vi "Main.vi"() -> ()   [LabVIEW 2016]
doc: "The myRIO Project template acquires acceleration data from the onboard accelerometer and displays the changes of acceleration values in a waveform chart."
uses:
  Project Custom Controls/IMU Data Cluster.ctl
  <vilib>/myRIO/Common/Instrument Driver Framework/myRIO v1.0/UART/vis/myRIO v1.0 Close UART.vi
  <vilib>/Instr/_visa.llb/VISA Configure Serial Port (Instr).vi
  <vilib>/myRIO/Common/Instrument Driver Framework/Utilities/vis/FPGA Ref Manager.vi
  <vilib>/myRIO/Common/Instrument Driver Framework/myRIO v1.0/myRIO v1.0 Reset FPGA.vi
  <vilib>/myRIO/Common/Instrument Driver Framework/myRIO v1.0/IRQ/vis/myRIO v1.0 IRQ Info FGV.vi
  <vilib>/myRIO/Common/Instrument Driver Framework/myRIO v1.0/IRQ/vis/myRIO v1.0 Timer IRQ Info FGV.vi
  <vilib>/myRIO/Common/Instrument Driver Framework/myRIO v1.0/IRQ/vis/myRIO v1.0 ISR Agent.vi
  <vilib>/myRIO/Instrument Drivers/Utilities/Utilities.lvlib
panel:
  in  "Roll Gains":T1
  in  "Roll":dbl min=0.0 max=0.08
  in  "Pitch":T1
  in  "Pitch":dbl min=0.0 max=0.08
  in  "Yaw Gains":T1
  in  "Yaw":dbl min=0.0 max=0.08
  in  "Start":bool
  out "Boolean 3":bool
  out "Boolean 2":bool
  out "Loop Iteration":dbl
  out "Waveform Chart":cluster{"Yaw":dbl, "Pitch":dbl, "Roll":dbl}(graph)
  in  "Stop":bool
  out "IMU Data Cluster":T2
  out "Boolean":bool
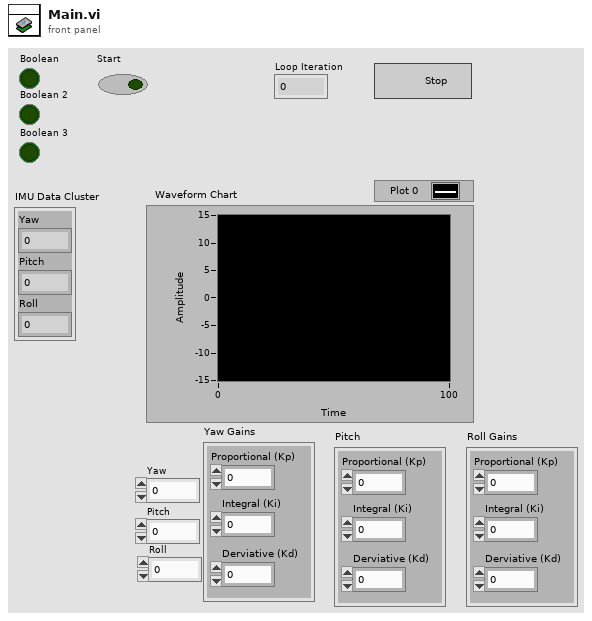
[diagram p1: front panel]
types:
  T1 = cluster{"Proportional (Kp)":dbl, "Integral (Ki)":dbl, "Derviative (Kd)":dbl}
  T2 = typedef "IMU Data Cluster.ctl" = cluster{"Yaw":dbl, "Pitch":dbl, "Roll":dbl}
  T3 = typedef "PWM.lvlib/PWM Reference.ctl" = cluster{"myRIO Reference":T4, "PWM Channels Enum":T8, "PWM Configuration":T9}
  T4 = typedef "myRIO Generic Hardware Reference.ctl" = cluster{"myRIO Model":T5, "myRIO Hardware Reference":T6}
  T5 = typedef "Hardware Version Enum.ctl" = enum16{"Unknown", "myRIO-1900", "myRIO-1950", "roboRIO", "NI ELVIS RIO CM"}
  T6 = typedef "myRIO v1.0 Reference.ctl" = cluster{"Generic FPGA Reference":T7, "Allow multiple opens":bool}
  T7 = typedef "Generic FPGA Reference.ctl" = refnum<k20>
  T8 = typedef "PWM Channels Enum.ctl" = enum16{"Not Connected", "C/PWM0", "C/PWM1", "A/PWM0", "A/PWM1", "A/PWM2", "B/PWM0", "B/PWM1", "B/PWM2", "PWM/PWM0", "PWM/PWM1", "PWM/PWM2", "PWM/PWM3", "PWM/PWM4", "PWM/PWM5", "PWM/PWM6", "PWM/PWM7", "PWM/PWM8", "PWM/PWM9"}
  T9 = typedef "PWM.lvlib/PWM Configuration.ctl" = cluster{"Frequency":dbl, "Duty Cycle":dbl}
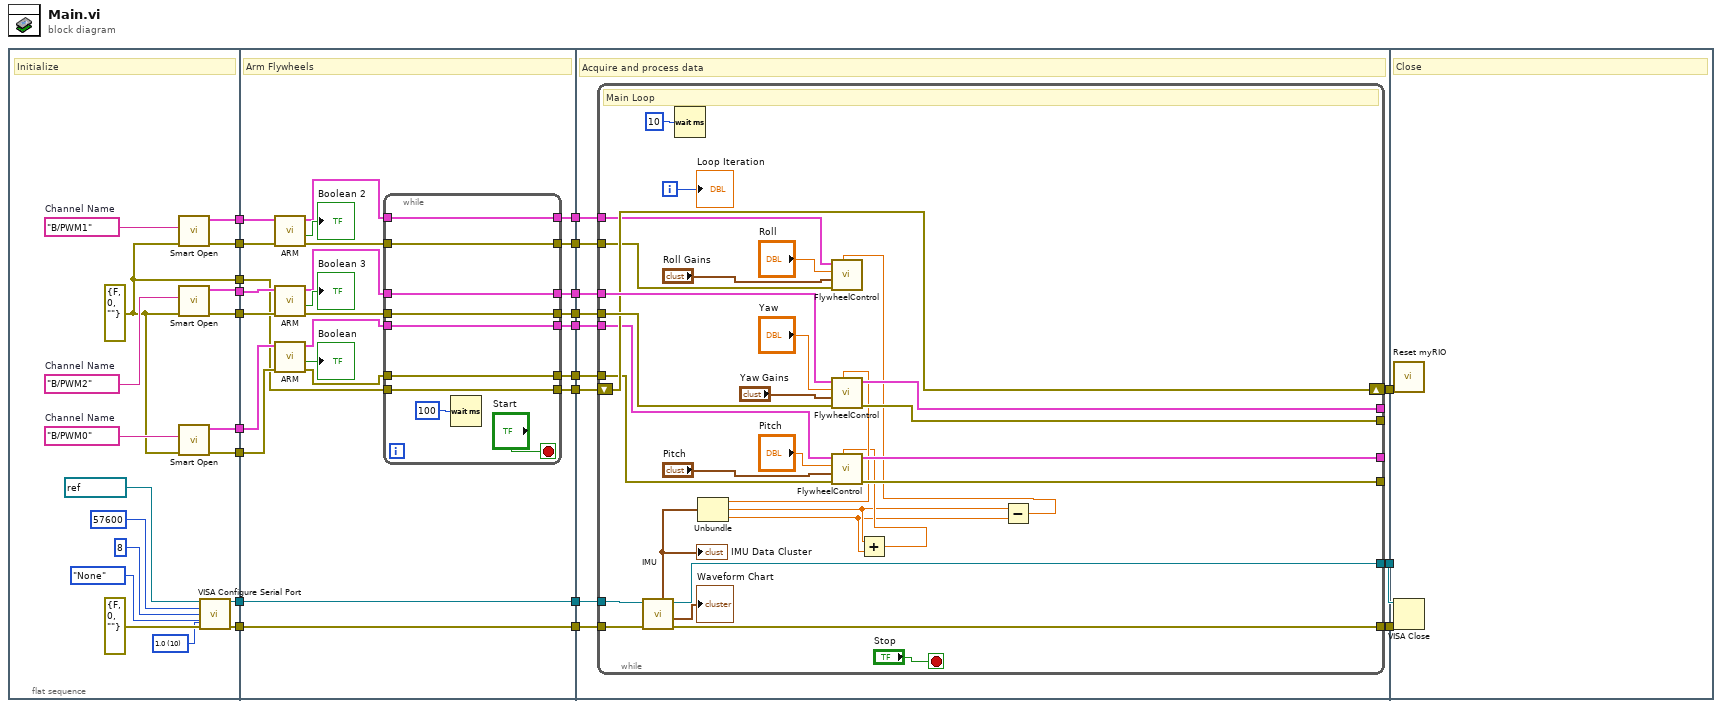
[diagram p0: block diagram]
diagram:
  n1 = flat-sequence {
    tunnel: [w34] -> w20
    tunnel: [w39] -> w19
    tunnel: [w38] -> w18
    tunnel: [w33] -> w17
    tunnel: [w32] -> w16
    tunnel: [w31] -> w15
    tunnel: [w30] -> w14
    tunnel: [w23] -> w5
    tunnel: [w22] -> w3
    tunnel: w20 -> [w55]
    tunnel: w19 -> [w64]
    tunnel: w18 -> [w63]
    tunnel: w17 -> [w62]
    tunnel: w16 -> [w61]
    tunnel: w15 -> [w60]
    tunnel: w14 -> [w59]
    tunnel: [w50] -> w13
    tunnel: [w48] -> w12
    tunnel: [w46] -> w11
    tunnel: [w44] -> w10
    tunnel: [w54] -> w9
    tunnel: [w52] -> w8
    tunnel: [w42] -> w7
    tunnel: [w41] -> w6
    tunnel: w5 -> [w41]
    tunnel: [w40] -> w4
    tunnel: w3 -> [w40]
    tunnel: [w85] -> w21
    tunnel: w13 -> [w84]
    tunnel: w12 -> [w83]
    tunnel: w11 -> [w82]
    tunnel: w10 -> [w81]
    tunnel: w9 -> [w78]
    tunnel: w8 -> [w80]
    tunnel: w7 -> [w79]
    tunnel: w6 -> [w76]
    tunnel: w4 -> [w77]
    tunnel: [w75] -> w2
    tunnel: [w74] -> w1
    tunnel: w21 -> [w119]
    tunnel: w2 -> [w118]
    tunnel: w1 -> [w117]
    frame #0 {
      w25 = u16 10 items=["1.0"=10, "1.5"=15, "2.0"=20] ("stop bits (10: 1 bit)")
      w35 = tag "B/PWM2"  # Channel Name
      w36 = tag "B/PWM1"  # Channel Name
      w37 = tag "B/PWM0"  # Channel Name
      w34 = errorcluster {"status"=FALSE, "code"=0, "source"=""} ("error in (no error)")
      # "Initialize"
      n2 = call <vilib>:"Smart Open.vi"("error in (no error)"=w34, "Channel Name"=w36) -> ("error out"=w32:errorcluster, "PWM Ref Out"=w33:T3)  [unwired: 8 in]
      n3 = call <vilib>:"Smart Open.vi"("error in (no error)"=w34, "Channel Name"=w35) -> ("error out"=w30:errorcluster, "PWM Ref Out"=w31:T3)  [unwired: 8 in]
      n4 = call <vilib>:"Smart Open.vi"("error in (no error)"=w34, "Channel Name"=w37) -> ("error out"=w38:errorcluster, "PWM Ref Out"=w39:T3)  [unwired: 8 in]
      n5 = call-poly "VISA Configure Serial Port"("VISA resource name"=refnum<visa-resource-name> "ASRL2::INSTR", "baud rate (9600)"=u32 57600, "data bits (8)"=u16 8, "parity (0:none)"=enum16{"None", "Odd", "Even", "Mark", "Space"}."None", "error in (no error)"=errorcluster {"status"=FALSE, "code"=0, "source"=""}, "stop bits (10: 1 bit)"=w25) -> ("VISA resource name out"=w23:refnum<visa-resource-name>, "error out"=w22:errorcluster)  [unwired: 8 in]
    }
    frame #1 {
      # "Arm Flywheels"
      n6 = call "ARM.vi"("error in (no error)"=w61, "PWM Ref in"=w62) -> ("error out"=w49:errorcluster, "Boolean"=→"Boolean 2":bool, "PWM Ref out"=w51:T3)  [unwired: 7 in]
      n7 = call "ARM.vi"("error in (no error)"=w59, "PWM Ref in"=w60) -> ("error out"=w45:errorcluster, "Boolean"=→"Boolean 3":bool, "PWM Ref out"=w47:T3)  [unwired: 7 in]
      n8 = call "ARM.vi"("error in (no error)"=w63, "PWM Ref in"=w64) -> ("error out"=w53:errorcluster, "Boolean"=→"Boolean":bool, "PWM Ref out"=w43:T3)  [unwired: 7 in]
      n9 = while {
        tunnel: w55 -> [w72]
        tunnel: [w72] -> w54
        tunnel: [w71] -> w52
        tunnel: w53 -> [w71]
        tunnel: [w70] -> w50
        tunnel: w51 -> [w70]
        tunnel: [w69] -> w48
        tunnel: w49 -> [w69]
        tunnel: [w68] -> w46
        tunnel: w47 -> [w68]
        tunnel: [w67] -> w44
        tunnel: w45 -> [w67]
        tunnel: [w65] -> w42
        tunnel: w43 -> [w65]
        stop <- "Start" stop-if-true
        n10 = Wait (ms)(milliseconds to wait=u32 100) -> ()  [unwired: 1 out]
      }
    }
    frame #2 {
      # "Acquire and process data"
      n11 = while {
        shift-right: [w106] -> w85
        shift-left: w78 -> [w106]
        tunnel: w80 -> [w101]
        tunnel: w79 -> [w100]
        tunnel: w84 -> [w99]
        tunnel: w83 -> [w98]
        tunnel: w82 -> [w114]
        tunnel: w81 -> [w113]
        tunnel: w77 -> [w112]
        tunnel: w76 -> [w111]
        tunnel: [w110] -> w75
        tunnel: [w109] -> w74
        tunnel: [w103] -> _
        tunnel: [w102] -> _
        tunnel: [w95] -> _
        tunnel: [w94] -> _
        i -> [w115]
        stop <- "Stop" stop-if-true
        # "Main Loop"
        n12 = call "IMU.vi"("error in (no error)"=w112, "VISA Refnum in"=w111) -> ("error out"=w109:errorcluster, "Waveform Chart"=→"Waveform Chart":cluster{"Yaw":dbl, "Pitch":dbl, "Roll":dbl}, "VISA Refnum out"=w110:refnum<visa-resource-name>, "IMU Data Cluster"=w91:T2)  [unwired: 5 in, 1 out]
        "IMU Data Cluster" <- w91
        n13 = Wait (ms)(milliseconds to wait=u32 10) -> ()  [unwired: 1 out]
        n14 = Unbundle(w91) -> ("Yaw"=w90:dbl, "Pitch"=w87:dbl, "Roll"=w86:dbl)
        n15 = call "FlywheelControl.vi"("Numeric"=w90, "error in (no error)"=w113, "Yaw Gains"="Yaw Gains", "Yaw"="Yaw", "PWM Ref in"=w114) -> ("error out"=w102:errorcluster, "PWM Ref Out"=w103:T3)  [unwired: 5 in]
        n16 = Add(x=w87, y=w86) -> (x+y=w89:dbl)
        n17 = call "FlywheelControl.vi"("Numeric"=w89, "error in (no error)"=w101, "Yaw Gains"="Pitch", "Yaw"="Pitch", "PWM Ref in"=w100) -> ("error out"=w94:errorcluster, "PWM Ref Out"=w95:T3)  [unwired: 5 in]
        n18 = Subtract(x=w87, y=w86) -> (x-y=w88:dbl)
        n19 = call "FlywheelControl.vi"("Numeric"=w88, "error in (no error)"=w98, "Yaw Gains"="Roll Gains", "Yaw"="Roll", "PWM Ref in"=w99) -> ()  [unwired: 5 in, 2 out]
        "Loop Iteration" <- w115
      }
    }
    frame #3 {
      # "Close"
      n20 = call <vilib>:"Reset myRIO.vi"("error in (no error)"=w119) -> ()  [unwired: 10 in, 1 out]
      n21 = VISA Close(VISA resource name=w118, error in (no error)=w117) -> ()  [unwired: 1 out]
    }
  }
